vi "FdxCmdRxSAPCreatePortCvi.vi"(8 "error in":errorcluster, 9 "SapCreateIn":T1, 11 "InstrumentHandle_port":u32) -> (0 "error out":errorcluster, 2 "UdpHandle":u32, 3 "InstrumentHandle_port":u32)   [LabVIEW 2020, in "AIM664LV.lvlib"]
doc: "Creates a port to receive data from a specified SAP connectionless port. This function can be used only, if receiver is not running. This function assumes that AiFdxCmdRxVLControl was previously called in order to enable a VL for reception. On this VL this function creates an AFDX SAP Rx-port."
uses:
  AIM664LV.lvlib
  AFDX_LibraryAdmin/FdxGlobalDllPath.vi
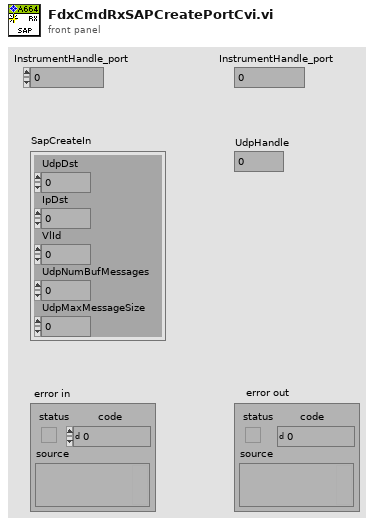
[diagram p1: front panel]
types:
  T1 = cluster{"UdpDst":u32, "IpDst":u32, "VlId":u32, "UdpNumBufMessages":u32, "UdpMaxMessageSize":u32}
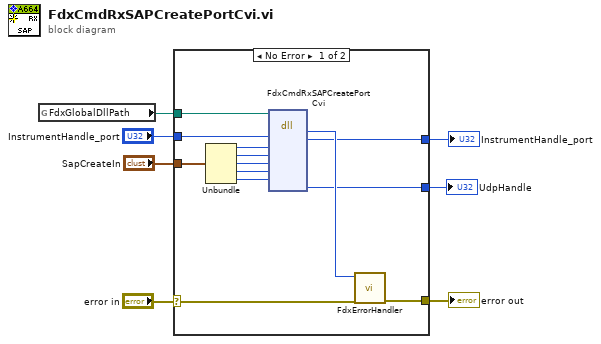
[diagram p0: block diagram]
diagram:
  n1 = global read "FdxGlobalDllPath.vi" "FdxGlobalDllPath"() -> (w5:path)
  n2 = case shown="No Error" "error in" {
    selector: "error in" -> [w19 w22]
    tunnel: [w20 w22] -> w7
    tunnel: w5 -> [w12 _]
    tunnel: "InstrumentHandle_port" -> [w11 w21]
    tunnel: [w10 w21] -> w3
    tunnel: "SapCreateIn" -> [w9 _]
    tunnel: [w8 _] -> w1
    frame No Error {
      n3 = Unbundle(w9) -> ("UdpDst"=w17:u32, "IpDst"=w16:u32, "VlId"=w15:u32, "UdpNumBufMessages"=w14:u32, "UdpMaxMessageSize"=w13:u32)
      n4 = dll-call lib="aim_fdx.19.dll" fn="FdxCmdRxSAPCreatePortCvi"(path in=w12, "InstrumentHandle"=w11, "UdpDst"=w17, "IpDst"=w16, "VlId"=w15, "UdpNumBufMessages"=w14, "UdpMaxMessageSize"=w13) -> ("status"=w18:i32, "InstrumentHandle"=w10:u32, "UdpHandle"=w8:u32)  [unwired: 7 in, 3 out]
      n5 = call "FdxErrorHandler.vi"("error in"=w19, "AIM Error"=w18) -> ("error out"=w20:errorcluster)  [unwired: 9 in]
    }
    frame Error {
    }
  }
  "error out" <- w7
  "InstrumentHandle_port" <- w3
  "UdpHandle" <- w1
